vi "Replace Mask Element.vi"(0 "Numeric":i16, 1 "Array":i16[][](array[numeric]), 11 "error in (no error)":errorcluster) -> (6 "concatenated string":string, 8 "row":i32, 10 "col":i32, 15 "error out":errorcluster)   [LabVIEW 2019]
panel:
  out "row total size":i32
  out "col total size":i32
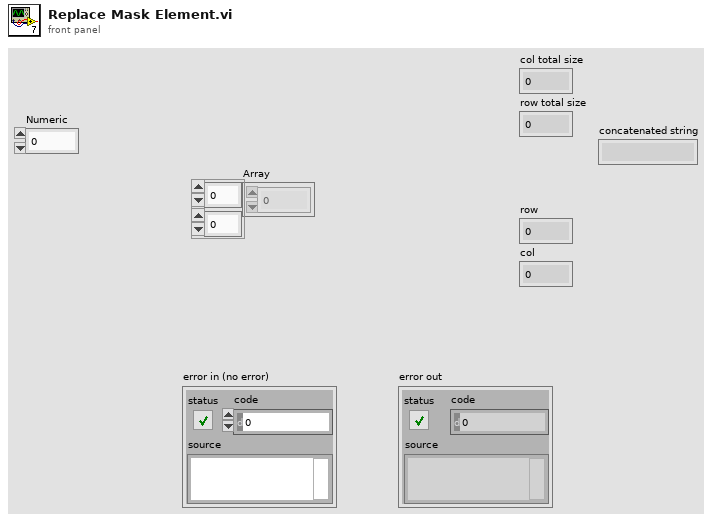
[diagram p1: front panel]
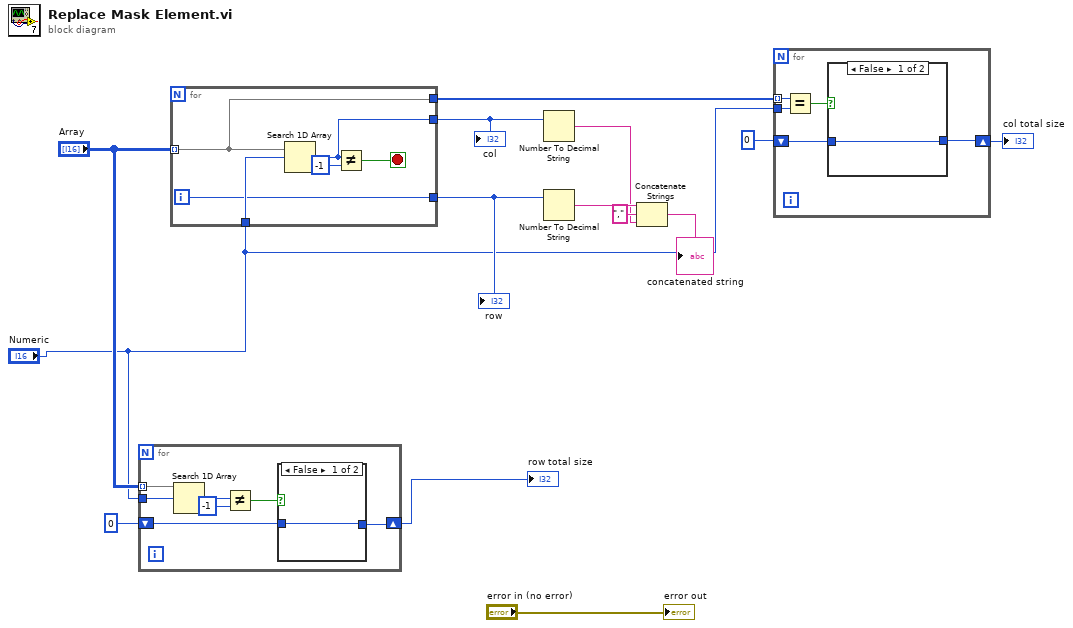
[diagram p0: block diagram]
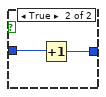
[diagram p2: hidden frame]
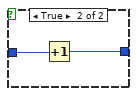
[diagram p3: hidden frame]
diagram:
  n1 = for {
    tunnel: "Array" -> [w21] mode=indexing
    tunnel: "Numeric" -> [w20]
    shift-right: [w15] -> w4
    shift-left: 0 -> [w16]
    n2 = Search 1D Array(1D array=w21, element=w20) -> (index of element=w19:i32)  [unwired: 1 in]
    n3 = Not Equal?(x=w19, y=-1) -> (x != y?=w17:bool)
    n4 = case shown="False" w17 {
      tunnel: w16 -> [w22 w24]
      tunnel: [w22 w23] -> w15
      frame False {
      }
      frame True {
        n5 = Increment(x=w24) -> (x+1=w23:i32)
      }
    }
  }
  "row total size" <- w4
  n6 = for {
    tunnel: "Array" -> [w25] mode=indexing
    tunnel: "Numeric" -> [w30]
    tunnel: [w27] -> w6
    tunnel: [w26] -> w7
    tunnel: [w25] -> w11
    i -> [w26]
    stop <- w28 stop-if-true
    n7 = Search 1D Array(1D array=w25, element=w30) -> (index of element=w27:i32)  [unwired: 1 in]
    n8 = Not Equal?(x=w27, y=-1) -> (x != y?=w28:bool)
  }
  "row" <- w7
  "col" <- w6
  n9 = Number To Decimal String(number=w6) -> (decimal integer string=w12:string)  [unwired: 1 in]
  n10 = Number To Decimal String(number=w7) -> (decimal integer string=w14:string)  [unwired: 1 in]
  n11 = Concatenate Strings(w14, "," ("string"), w12) -> (→"concatenated string":string)
  n12 = for {
    tunnel: w11 -> [w35] mode=indexing
    shift-right: [w31] -> w5
    shift-left: 0 -> [w32]
    tunnel: "Numeric" -> [w34]
    n13 = Equal?(x=w35, y=w34) -> (x = y?=w33:bool)
    n14 = case shown="False" w33 {
      tunnel: w32 -> [w36 w38]
      tunnel: [w36 w37] -> w31
      frame False {
      }
      frame True {
        n15 = Increment(x=w38) -> (x+1=w37:i32)
      }
    }
  }
  "col total size" <- w5
  "error out" <- "error in (no error)"
